vi "Put Timestamped Segment.vi"(0 "TreeNode in":refnum<class "TreeNode.lvclass">, 5 "Segment data":refnum<class "Data.lvclass">, 7 "Timestamps":i64[](array[numeric]), 11 "error in (no error)":errorcluster) -> (4 "TreeNode out":refnum<class "TreeNode.lvclass">, 15 "error out":errorcluster)   [LabVIEW 2015, in "MDSplus.lvlib" / "TreeNode.lvclass"]
doc: "Write a single row of timestamped data."
uses:
  <vilib>/MDSplus/Classes/Data_Class/TreeNode_Class/TreeNode.lvclass
  <vilib>/MDSplus/Classes/Data_Class/Data.lvclass
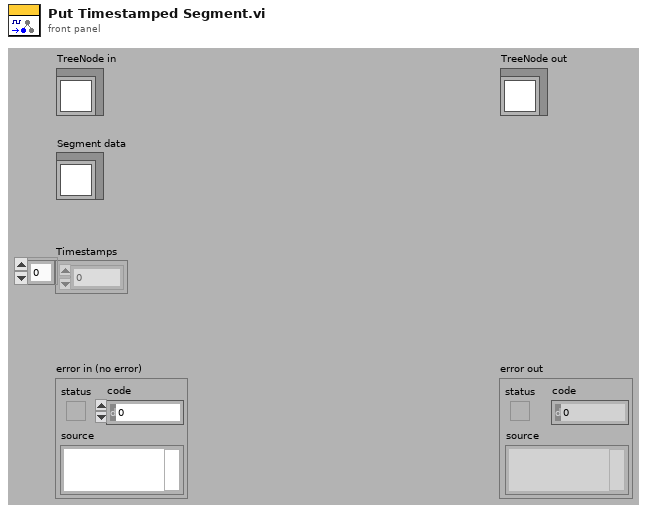
[diagram p1: front panel]
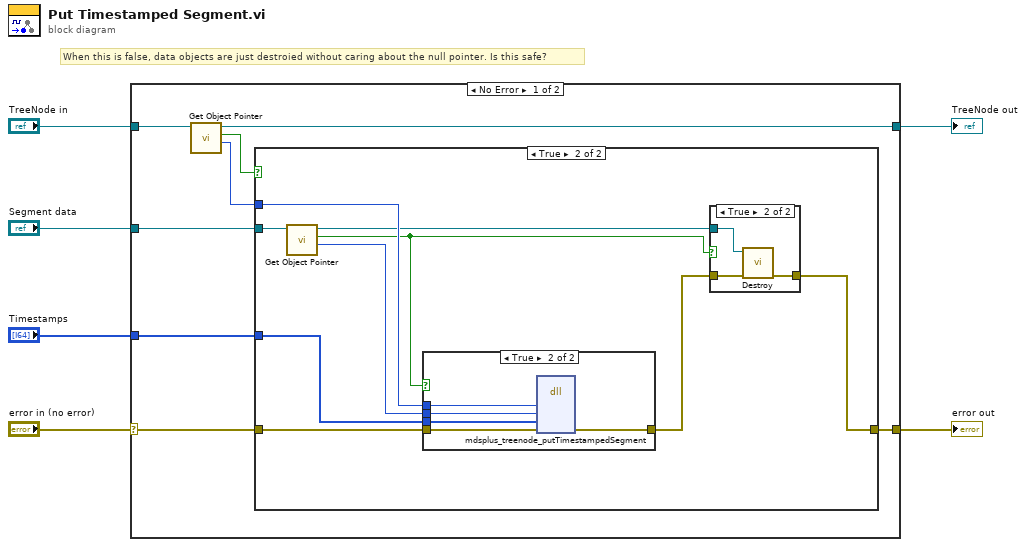
[diagram p0: block diagram]
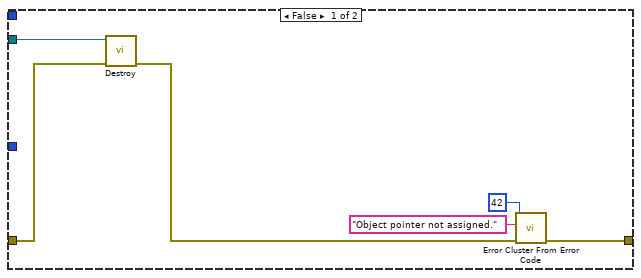
[diagram p2: hidden frame]
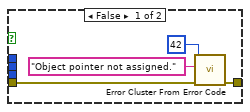
[diagram p4: hidden frame]
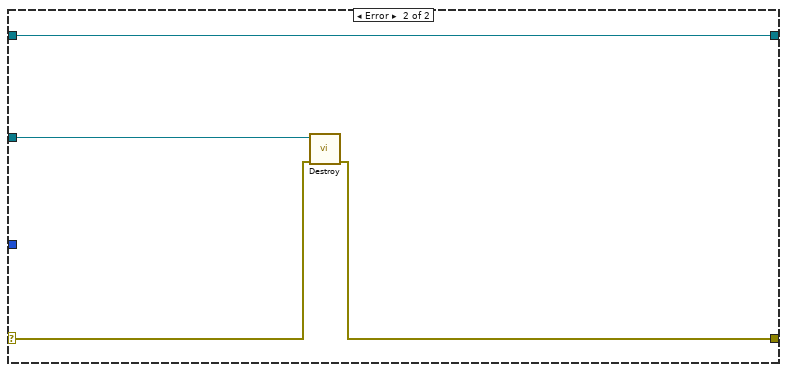
[diagram p5: hidden frame]
diagram:
  # "When this is false, data objects are just destroied without caring about the null pointer. Is this safe?"
  n1 = case shown="No Error" "error in (no error)" {
    selector: "error in (no error)" -> [w8 w44]
    tunnel: [w7 w43] -> w5
    tunnel: [w13 w46] -> w3
    tunnel: "TreeNode in" -> [w14 w46]
    tunnel: "Segment data" -> [w10 w45]
    tunnel: "Timestamps" -> [w9 _]
    frame No Error {
      n2 = call-dynamic "Get Object Pointer.vi"("Data in"=w14) -> ("Object Pointer"=w12:i64, "Assigned object pointer?"=w11:bool, "Data out"=w13:refnum<class "TreeNode.lvclass">)  [unwired: 8 in]
      n3 = case shown="True" w11 {
        tunnel: w10 -> [w17 w29]
        tunnel: w12 -> [_ w27]
        tunnel: w8 -> [w16 w26]
        tunnel: [w18 w21] -> w7
        tunnel: w9 -> [_ w23]
        frame False {
          n4 = call-dynamic "Destroy.vi"("error in (no error)"=w16, "Data in"=w17) -> ("error out"=w15:errorcluster)  [unwired: 9 in]
          n5 = call <vilib>:"Error Cluster From Error Code.vi"("error in (no error)"=w15, "error message (\"\")"="Object pointer not assigned." ("error message (\"\")"), "error code (0)"=42) -> ("error out"=w18:errorcluster)  [unwired: 6 in]
        }
        frame True {
          n6 = call-dynamic "Get Object Pointer.vi"("Data in"=w29) -> ("Object Pointer"=w28:i64, "Assigned object pointer?"=w22:bool, "Data out"=w24:refnum<class "Data.lvclass">)  [unwired: 8 in]
          n7 = case shown="True" w22 {
            tunnel: w28 -> [_ w41]
            tunnel: w27 -> [_ w42]
            tunnel: w26 -> [w34 w39]
            tunnel: [w35 w38] -> w25
            tunnel: w23 -> [_ w40]
            frame False {
              n8 = call <vilib>:"Error Cluster From Error Code.vi"("error in (no error)"=w34, "error message (\"\")"="Object pointer not assigned." ("error message (\"\")"), "error code (0)"=42) -> ("error out"=w35:errorcluster)  [unwired: 6 in]
            }
            frame True {
              n9 = dll-call lib="MDSobjectsLVShr" fn="mdsplus_treenode_putTimestampedSegment"("lvTreeNodePtr"=w42, "lvArrayPtrIn"=w41, "lvLngArrHdlIn"=w40, "error"=w39) -> ("error"=w38:errorcluster)  [unwired: 7 in, 2 out]
            }
          }
          n10 = case shown="True" w22 {
            tunnel: w25 -> [w30 w33]
            tunnel: w24 -> [_ w32]
            tunnel: [w30 w31] -> w21
            frame False {
            }
            frame True {
              n11 = call-dynamic "Destroy.vi"("error in (no error)"=w33, "Data in"=w32) -> ("error out"=w31:errorcluster)  [unwired: 9 in]
            }
          }
        }
      }
    }
    frame Error {
      n12 = call-dynamic "Destroy.vi"("error in (no error)"=w44, "Data in"=w45) -> ("error out"=w43:errorcluster)  [unwired: 9 in]
    }
  }
  "error out" <- w5
  "TreeNode out" <- w3
